vi "Scale 32 Bit.vi"(8 "error in (no error)":errorcluster, 11 "Data Scaling in":refnum<class "Data Scaling.lvclass">) -> (0 "error out":errorcluster, 3 "Data Scaling out":refnum<class "Data Scaling.lvclass">)   [LabVIEW 2020, in "Unit Tests.lvlib" / "Data Scaling.lvclass"]
uses:
  Data Scaling.lvclass
  Frames & Messages/TypeDefs/Scaling Information.ctl
  <vilib>/addons/_JKI Toolkits/Caraya/classes/Test/Test.lvclass
  <vilib>/addons/_JKI Toolkits/Caraya/classes/Assert/Assert.lvclass
  BCI-1553 API.lvlib
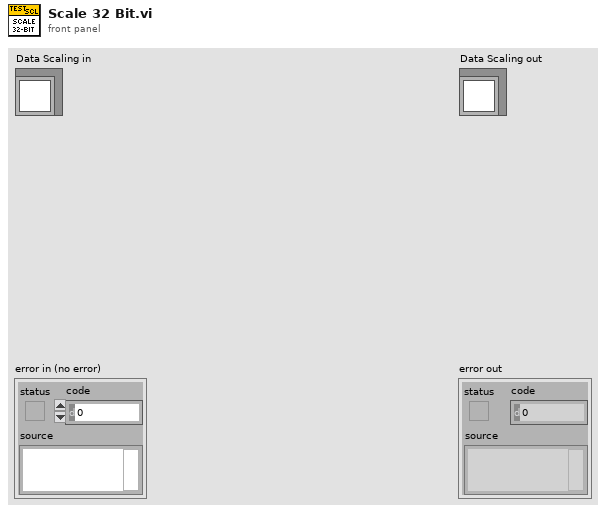
[diagram p1: front panel]
types:
  T1 = typedef "BCI-1553 API.lvlib/Scaling Information.ctl" = cluster{"Bit Offset":i32, "Bit Count":i32, "LSB Resolution":dbl, "2's Complement":bool, "Big Endian":bool, "Sign Bit":bool}
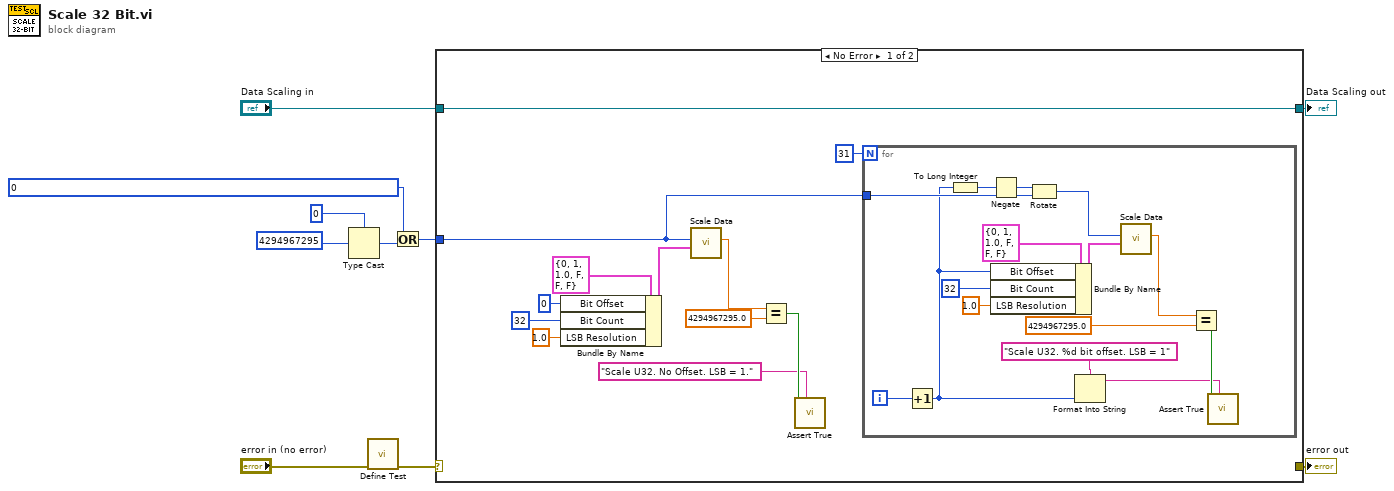
[diagram p0: block diagram]
diagram:
  n1 = Type Cast(type=u64 0 ("unsigned 64bit integer"), x=u32 4294967295 ("unsigned 8bit integer")) -> (*(type *) &x=w2:u64)
  n2 = call <vilib>:"Define Test.vi"("error in (no error)"="error in (no error)") -> ("error out"=w6:errorcluster)  [unwired: 9 in, 1 out]
  n3 = Or(x=u64 0 ("Raw Value"), y=w2) -> (x .or. y?=w5:u64)
  n4 = case shown="No Error" w6 {
    selector: w6 -> [_ w39]
    tunnel: [_ w39] -> w10
    tunnel: [w22 w38] -> w8
    tunnel: "Data Scaling in" -> [w22 w38]
    tunnel: w5 -> [w12 _]
    frame No Error {
      n5 = Bundle By Name(cluster=T1 {"Bit Offset"=0, "Bit Count"=1, "LSB Resolution"=1.0, "2's Complement"=FALSE, "Big Endian"=FALSE, "Sign Bit"=FALSE} ("Scaling Info"), "Bit Offset"=0, "Bit Count"=32, "LSB Resolution"=1.0) -> (w17:T1)
      n6 = call "Scale Data.vi"("Scaling Info"=w17, "Raw Value"=w12) -> ("Scaled Value"=w16:dbl)  [unwired: 8 in, 1 out]
      n7 = Equal?(x=w16, y=4294967295.0) -> (x = y?=w14:bool)
      n8 = call <vilib>:"Assert True.vi"("Label"="Scale U32. No Offset. LSB = 1.", "True?"=w14) -> ()  [unwired: 8 in, 2 out]
      n9 = for {
        N: 31 -> [_]
        tunnel: w12 -> [w31]
        i -> [w29]
        n10 = Increment(x=w29) -> (x+1=w26:i32)
        n11 = To Long Integer(number=w26) -> (32bit integer=w23:i32)
        n12 = Negate(x=w23) -> (-x=w25:i32)
        n13 = Bundle By Name(cluster=T1 {"Bit Offset"=0, "Bit Count"=1, "LSB Resolution"=1.0, "2's Complement"=FALSE, "Big Endian"=FALSE, "Sign Bit"=FALSE} ("Scaling Info"), "Bit Offset"=w26, "Bit Count"=32, "LSB Resolution"=1.0) -> (w35:T1)
        n14 = Rotate(1:w31, 2:w25) -> (0:w30:u64)
        n15 = Format Into String(format string="Scale U32. %d bit offset. LSB = 1" ("Label"), w26) -> (resulting string=w27:string)  [unwired: 2 in, 1 out]
        n16 = call "Scale Data.vi"("Scaling Info"=w35, "Raw Value"=w30) -> ("Scaled Value"=w36:dbl)  [unwired: 8 in, 1 out]
        n17 = Equal?(x=w36, y=4294967295.0) -> (x = y?=w37:bool)
        n18 = call <vilib>:"Assert True.vi"("Label"=w27, "True?"=w37) -> ()  [unwired: 8 in, 2 out]
      }
    }
    frame Error {
    }
  }
  "error out" <- w10
  "Data Scaling out" <- w8
